vi "Push_Data_Client.vi"(5 "Archive File?":bool, 6 "application reference":refnum<vi>, 7 "error in (no error)":errorcluster, 8 "Running on Server?":bool, 10 "Path of File relative to EnFlo Data Root":path) -> (0 "error out":errorcluster)   [LabVIEW 2011]
uses:
  Anemometry/Anemometry Sub Vis/Globals/Constants_global.vi
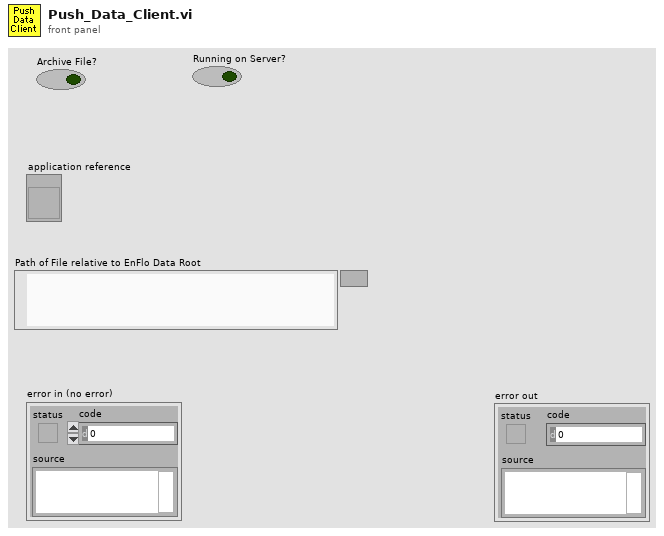
[diagram p1: front panel]
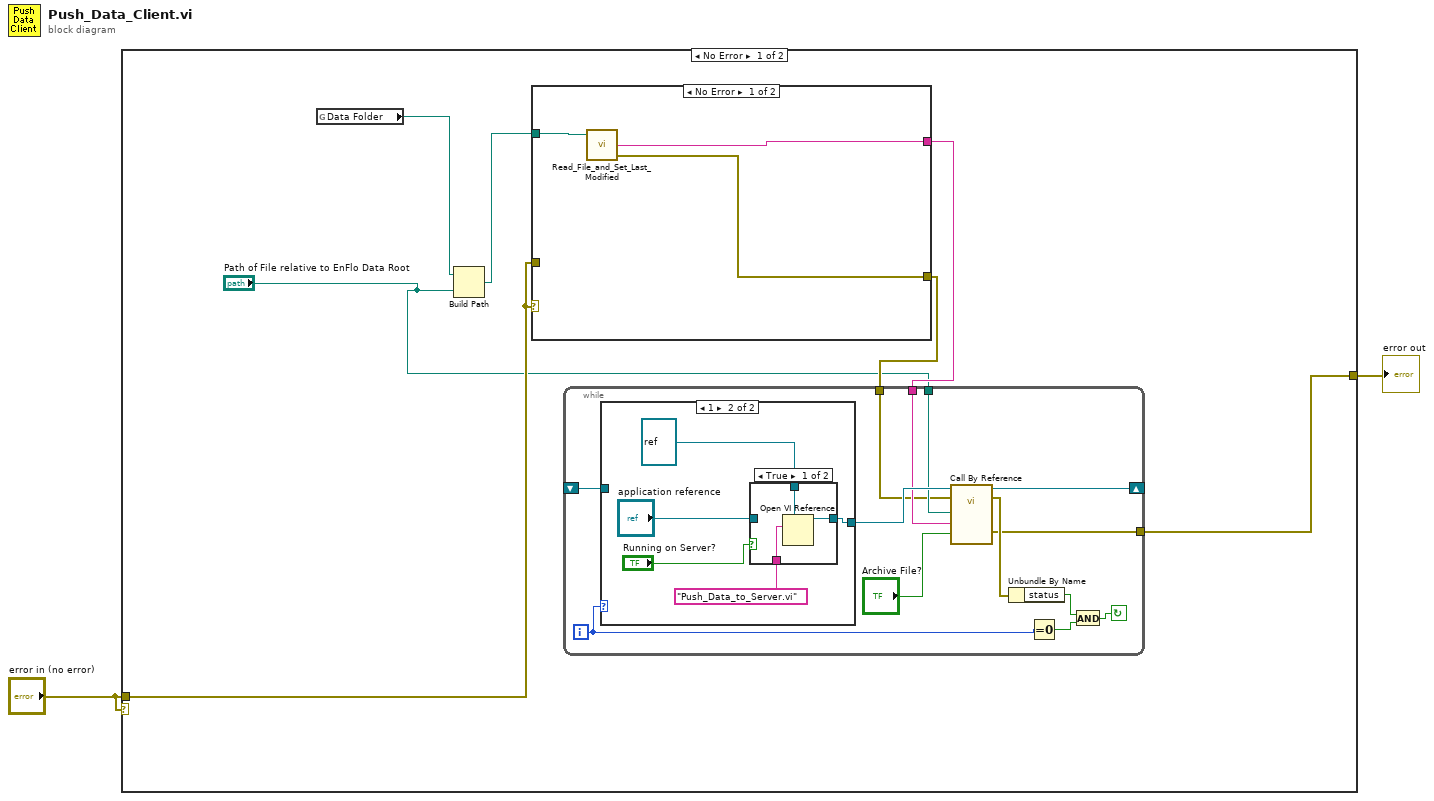
[diagram p0: block diagram]
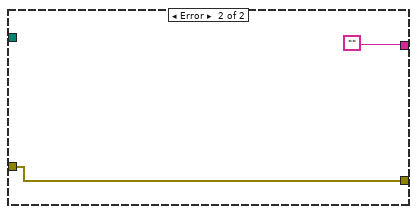
[diagram p2: hidden frame]
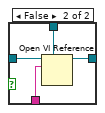
[diagram p4: hidden frame]
diagram:
  n1 = case shown="No Error" "error in (no error)" {
    tunnel: [w3 w41] -> w2
    tunnel: "error in (no error)" -> [w8 w41]
    frame No Error {
      n2 = global read "Constants_global.vi" "Data Folder"() -> (w9:path)
      n3 = Build Path(base path=w9, name or relative path="Path of File relative to EnFlo Data Root") -> (appended path=w7:path)
      n4 = case shown="No Error" w8 {
        tunnel: w7 -> [w11 _]
        tunnel: [w12 ""] -> w5
        tunnel: [w10 w13] -> w6
        tunnel: w8 -> [_ w13]
        frame No Error {
          n5 = call "Read_File_and_Set_Last_Modified.vi"("file path"=w11) -> ("error out"=w10:errorcluster, "string"=w12:string)  [unwired: 2 in, 1 out]
        }
        frame Error {
        }
      }
      n6 = while {
        shift-right: [w25] -> _
        shift-left: _ -> [w27]
        tunnel: "Path of File relative to EnFlo Data Root" -> [w20]
        tunnel: w5 -> [w19]
        tunnel: [w17] -> w3
        tunnel: w6 -> [w15]
        i -> [w24]
        stop <- w21 continue-if-true
        n7 = case shown="1" w24 {
          tunnel: w27 -> [w28 _]
          tunnel: [w28 w33] -> w26
          frame 0, Default {
          }
          frame 1 {
            n8 = case shown="True" "Running on Server?" {
              tunnel: [w36 w40] -> w33
              tunnel: "application reference" -> [_ w39]
              tunnel: refnum<vi> refnum ("Push Data Server") -> [w35 w38]
              tunnel: "Push_Data_to_Server.vi" -> [w34 w37]
              frame True {
                n9 = Open VI Reference(type specifier VI Refnum (for type only)=w35, vi path=w34) -> (vi reference=w36:refnum<vi>)  [unwired: 2 in, 3 out]
              }
              frame False {
                n10 = Open VI Reference(type specifier VI Refnum (for type only)=w38, application reference (local)=w39, vi path=w37) -> (vi reference=w40:refnum<vi>)  [unwired: 1 in, 3 out]
              }
            }
          }
        }
        n11 = call-by-ref "?"(reference=w26, error in=w15, "Archive File?"="Archive File?", "Zip String"=w19, "Relative Path"=w20) -> (reference out=w25:refnum<vi>, error out=w18:errorcluster, "error out"=w17:errorcluster)  [unwired: 1 in]
        n12 = Unbundle By Name(w18) -> ("status"=w22:bool)
        n13 = Equal To 0?(x=w24) -> (x = 0?=w23:bool)
        n14 = And(x=w22, y=w23) -> (x .and. y?=w21:bool)
      }
    }
    frame Error {
    }
  }
  "error out" <- w2
